vi "eCompass.vi"() -> ()   [LabVIEW 2019]
uses:
  Program Files (x86)/National Instruments/LabVIEW 2019/examples/Instrument IO/Serial/support/Serial - Settings.ctl
  <vilib>/Instr/_visa.llb/VISA Configure Serial Port (Instr).vi
panel:
  in  "Stop":bool
  out "Response":string
  out "bytes read":u32
  in  "Serial Settings":T1={"baud rate"=19200, "data bits"=8, "parity"=enum."None", "stop bits"=10, "flow control"=0} {"flow control" items=["None"=0, "XON/XOFF"=1, "RTS/CTS"=2, "DTR/DSR"=4]; "stop bits" items=["1.0"=10, "1.5"=15, "2.0"=20]; "data bits" min=5 max=8 step=1; "baud rate" items=["75"=75, "110"=110, "134"=134, "150"=150, "300"=300, "600"=600, "1200"=1200, "1800"=1800, "2400"=2400, "4800"=4800, "7200"=7200, "9600"=9600, "14400"=14400, "19200"=19200, "28800"=28800, "38400"=38400, "56000"=56000, "57600"=57600, "115200"=115200, "128000"=128000, "230400"=230400]}
  in  "delay before read (ms)":u32=50
  in  "Com Port":refnum<visa-resource-name>="COM3"
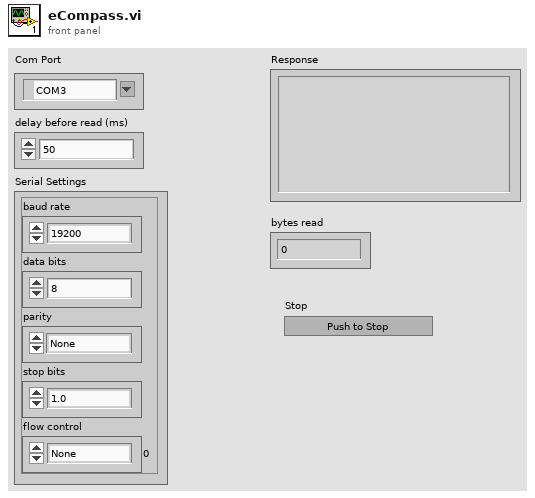
[diagram p1: front panel]
types:
  T1 = typedef "Serial - Settings.ctl" = cluster{"baud rate":u32, "data bits":u16, "parity":enum16{"None", "Odd", "Even", "Mark", "Space"}, "stop bits":u16, "flow control":u16}
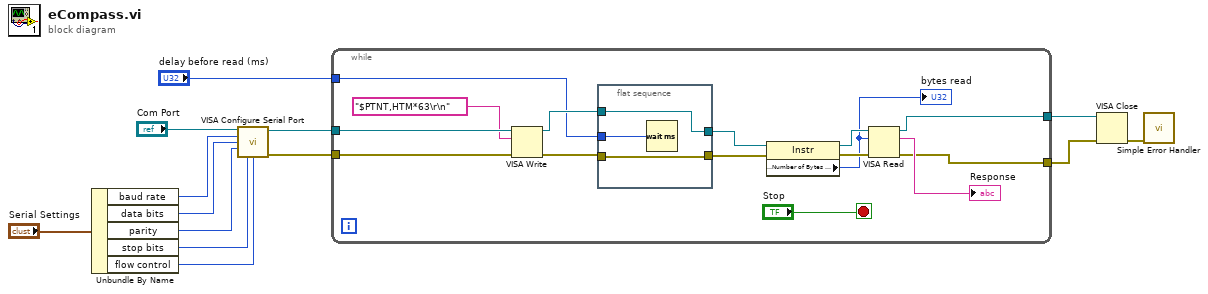
[diagram p0: block diagram]
diagram:
  n1 = Unbundle By Name("Serial Settings") -> ("baud rate"=w8:u32, "data bits"=w7:u16, "parity"=w6:enum16{"None", "Odd", "Even", "Mark", "Space"}, "stop bits"=w5:u16, "flow control"=w4:u16)
  n2 = call-poly "VISA Configure Serial Port"("VISA resource name"="Com Port", "baud rate (9600)"=w8, "data bits (8)"=w7, "parity (0:none)"=w6, "stop bits (10: 1 bit)"=w5, "flow control (0:none)"=w4) -> ("VISA resource name out"=w11:refnum<visa-resource-name>, "error out"=w12:errorcluster)  [unwired: 3 in, 5 out]
  n3 = while {
    tunnel: w12 -> [w28]
    tunnel: w11 -> [w27]
    tunnel: "delay before read (ms)" -> [w22]
    tunnel: [w16] -> w3
    tunnel: [w15] -> w2
    stop <- "Stop" stop-if-true
    n4 = VISA Write(VISA resource name=w27, write buffer="$PTNT,HTM*63\r\n" ("Command"), error in (no error)=w28) -> (VISA resource name out=w24:refnum<visa-resource-name>, error out=w26:errorcluster)  [unwired: 1 out]
    n5 = flat-sequence {
      tunnel: w26 -> [w30]
      tunnel: [w30] -> w25
      tunnel: w24 -> [w29]
      tunnel: [w29] -> w23
      tunnel: w22 -> [w31]
      frame #0 {
        n6 = Wait (ms)(milliseconds to wait=w31) -> ()  [unwired: 1 out]
      }
    }
    n7 = property class="Instr"(reference=w23, error in=w25) -> (reference out=w20:refnum<visa-resource-name>, error out=w19:errorcluster, "Serial Settings:Number of Bytes at Serial Port"=w17:u32)
    "bytes read" <- w17
    n8 = VISA Read(VISA resource name=w20, byte count=w17, error in (no error)=w19) -> (VISA resource name out=w15:refnum<visa-resource-name>, read buffer=→"Response":string, error out=w16:errorcluster)  [unwired: 1 out]
  }
  n9 = VISA Close(VISA resource name=w2, error in (no error)=w3) -> (error out=w1:errorcluster)
  n10 = call <vilib>:"Simple Error Handler.vi"("error in (no error)"=w1) -> ()  [unwired: 1 in, 8 out]
